vi "Util_DispWeightedWaypoint_Eng_To_WeightedWaypoint_SI.vi"(11 "DisplayWeightedWayPoints_ENG":T4[](array[typedef]) {"WEIGHT" format="%13.3f"; "ANGLE" format="%13.3f"; "Y" format="%13.3f"; "X" format="%13.3f"}) -> (3 "WeightedWayPoints_SI":T1[](array[typedef]) {"SCALAR" format="%14.3f"; "ROTATION"."SIN" format="%13.4f"; "ROTATION"."COS" format="%13.4f"; "ROTATION"."VALUE" format="%13.4f"; "TRANSLATION"."Y" format="%14.3f"; "TRANSLATION"."X" format="%14.3f"})   [LabVIEW 2019, in "Trajectory_Library.lvlib"]
doc: "Utility function to convert utility (displayable) weighted waypoints from Inches, degrees to meters, radians. All the normal trajectory functions expect the units to be in meters, radians (unless otherwise specified).\n\nThis then converted from the utility weighted waypoints, which are good for putting on front panels, to normal weighted waypoints that are used by the trajectory generation functions."
uses:
  Trajectory_Library.lvlib
  DISPLAY_WEIGHTED_WAYPOINT.ctl
  WEIGHTED_WAYPOINT.ctl
  TRANSLATION2D.ctl
  ROTATION2D.ctl
  Translation2d_Create.vi
  Rotation2d_CreateAngle.vi
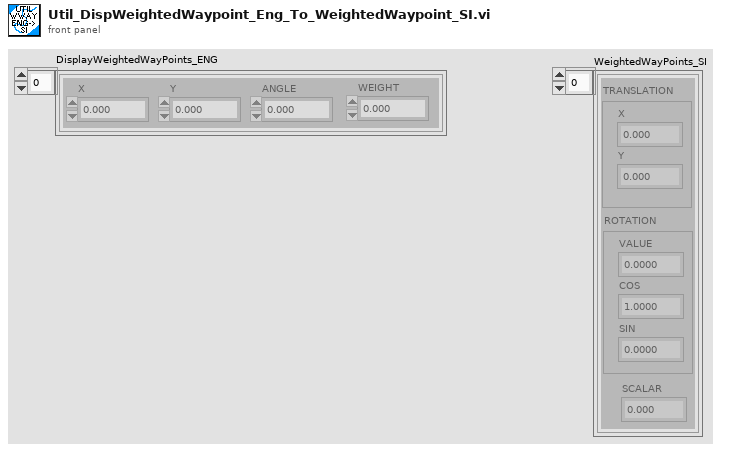
[diagram p1: front panel]
types:
  T1 = typedef "Trajectory_Library.lvlib/WEIGHTED_WAYPOINT.ctl" = cluster{"TRANSLATION":T2, "ROTATION":T3, "SCALAR":dbl}
  T2 = typedef "Trajectory_Library.lvlib/TRANSLATION2D.ctl" = cluster{"X":dbl, "Y":dbl}
  T3 = typedef "Trajectory_Library.lvlib/ROTATION2D.ctl" = cluster{"VALUE":dbl, "COS":dbl, "SIN":dbl}
  T4 = typedef "Trajectory_Library.lvlib/DISPLAY_WEIGHTED_WAYPOINT.ctl" = cluster{"X":dbl, "Y":dbl, "ANGLE":dbl, "WEIGHT":dbl}
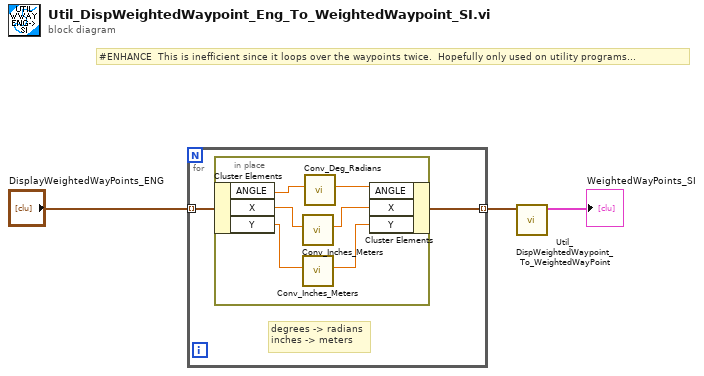
[diagram p0: block diagram]
diagram:
  # "#ENHANCE  This is inefficient since it loops over the waypoints twice.  Hopefully only used on utility programs..."
  n1 = for {
    tunnel: "DisplayWeightedWayPoints_ENG" -> [w5] mode=indexing
    tunnel: [w4] -> w2 mode=indexing
    # "degrees -> radians\ninches -> meters"
    n2 = in-place {
      n3 = in-place-cluster #1(w5) -> ("ANGLE"=w6:dbl, "X"=w11:dbl, "Y"=w9:dbl)
      n4 = call "Conv_Inches_Meters.vi"("INCH"=w11) -> ("Meters"=w10:dbl)  [unwired: 10 in]
      n5 = call "Conv_Inches_Meters.vi"("INCH"=w9) -> ("Meters"=w8:dbl)  [unwired: 10 in]
      n6 = call "Conv_Deg_Radians.vi"("Degress"=w6) -> ("Radians"=w7:dbl)  [unwired: 10 in]
      n7 = in-place-cluster #1("ANGLE"=w7, "X"=w10, "Y"=w8) -> (w4:T4)
    }
  }
  n8 = call "Util_DispWeightedWaypoint_To_WeightedWayPoint.vi"("DisplayWeightedWayPoints"=w2) -> ("WeightedWayPoints"=→"WeightedWayPoints_SI":T1[])  [unwired: 10 in]
